vi "Halvorsen_2D_Lyapunov.vi"(11 "Initial Conditions":ext[](array[numeric])=[0.1, 0.0, 0.1]) -> ()   [LabVIEW 2016]
panel:
  out "Elapsed Time, s.":dbl
  out "Lyapunov":ext[][](graph)
  in  "Initial Conditions Inc":ext[](array[numeric])=[1e-10, 1e-10, 1e-10]
  in  "X_Inc":dbl[](array[numeric])=[0.02, 0.0, 0.0]
  in  "Final_X":dbl=0.35
  in  "Param_X":i32
  in  "Param_Y":i32=1
  in  "Final Y":dbl=0.35
  in  "Y_Inc":dbl[](array[numeric])=[0.0, 0.02, 0.0]
  in  "Parameter_Vector":ext[](array[numeric])=[0.01, 0.01, 0.1]
  out "Current_Param":ext[](array[numeric])=[0.01, 0.29000000000000000582, 0.1]
  in  "Время, с":ext=300.0
  in  "Hmin":ext=0.00099999999999999999996
  in  "Hmax":ext=1.0
  in  "tolerance":ext=1e-12
  in  "Шаг h, с":ext=0.01
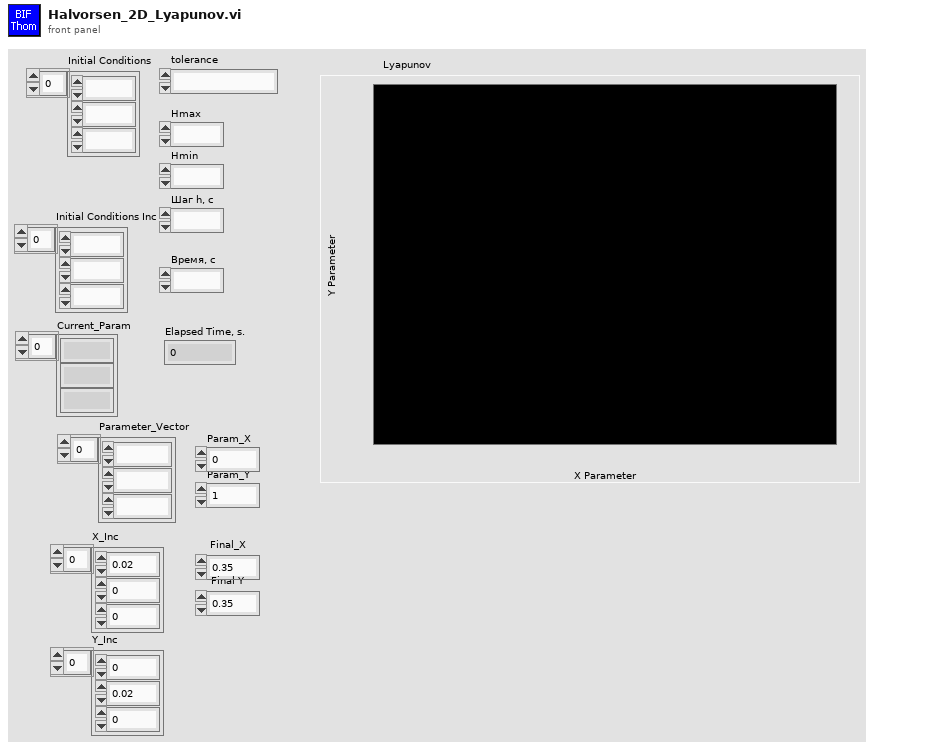
[diagram p1: front panel]
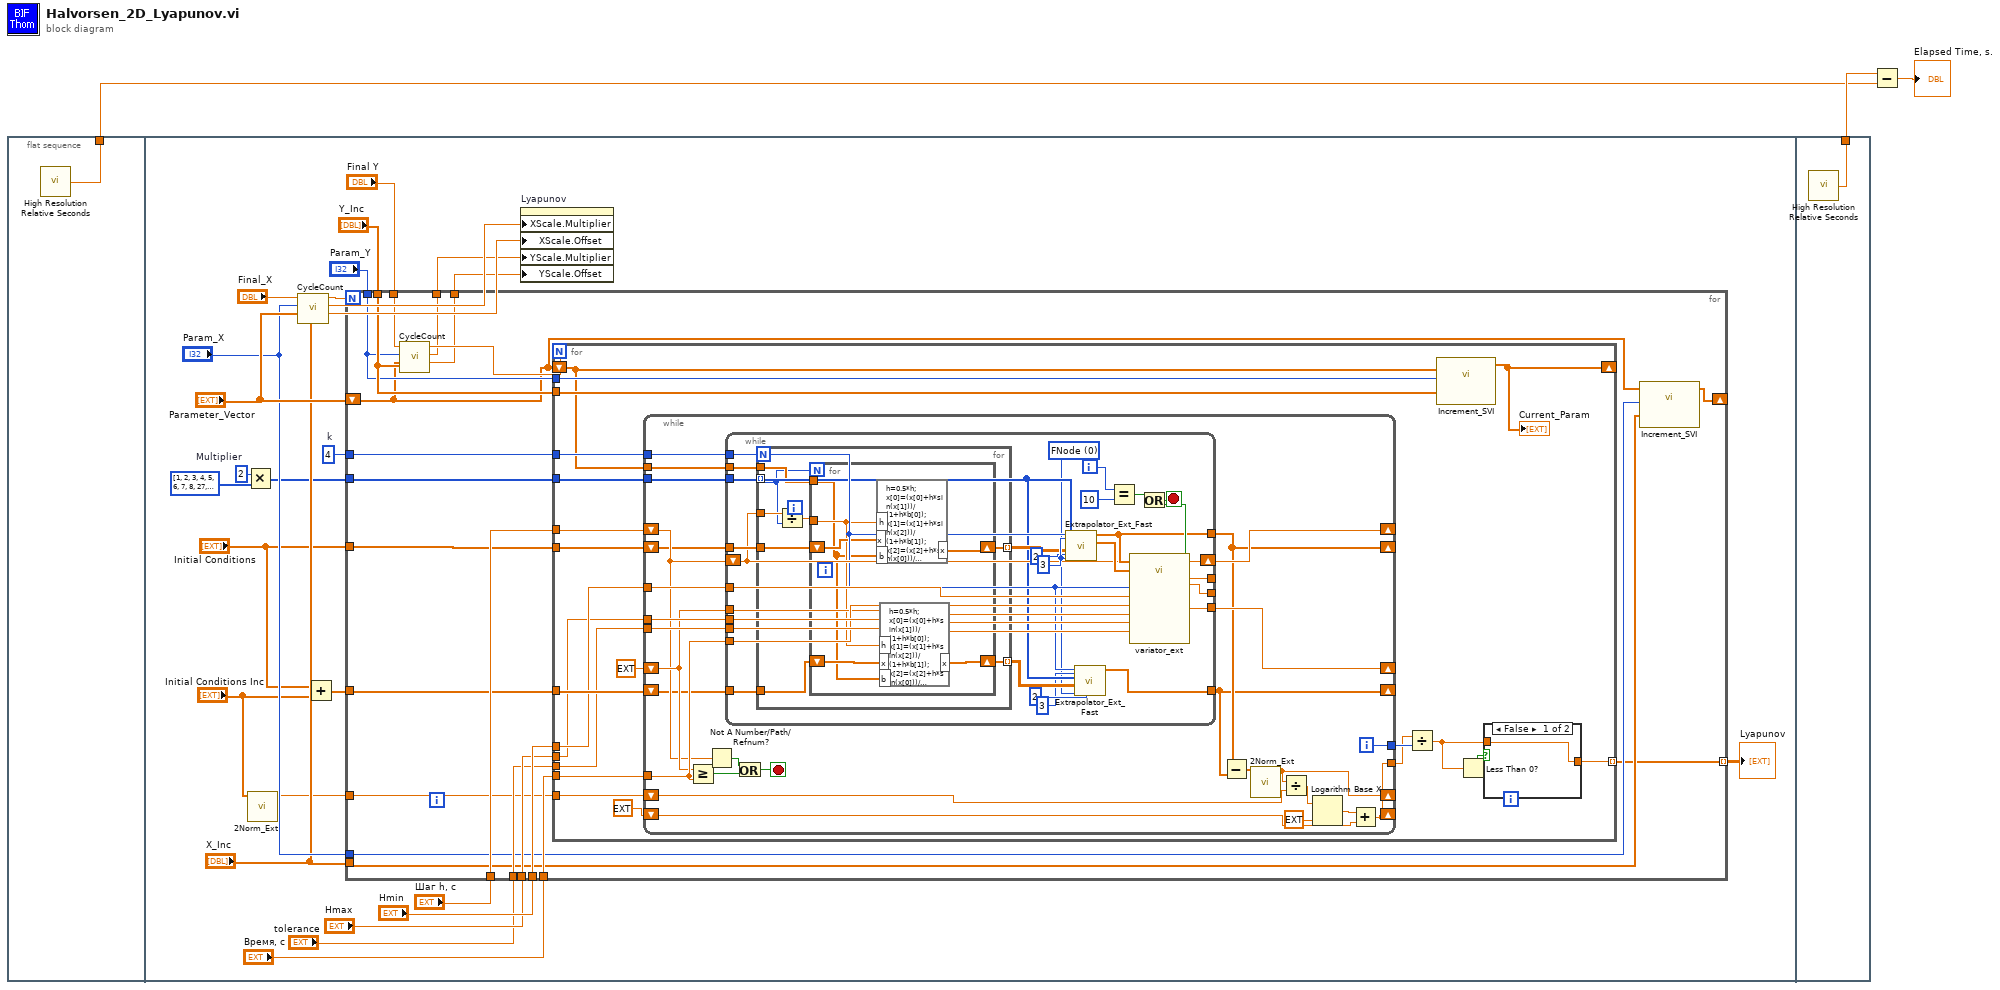
[diagram p0: block diagram]
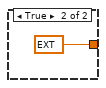
[diagram p2: hidden frame]
diagram:
  n1 = flat-sequence {
    tunnel: [w4] -> w2
    tunnel: [w145] -> w3
    frame #0 {
      n2 = call <vilib>:"High Resolution Relative Seconds.vi"() -> ("relative seconds"=w4:dbl)
    }
    frame #1 {
      w10 = 4  # k
      w17 = 2  # Multiplier
      n3 = Multiply(x=w17, y=i32[] [1, 2, 3, 4, 5, 6, 7, 8, 27, 30, 33] ("n")) -> (x*y=w15:i32[])
      n4 = call "2Norm_Ext.vi"("Input vector"="Initial Conditions Inc") -> ("2 Norm"=w13:ext)  [unwired: 10 in]
      n5 = call "CycleCount.vi"("Increment_Vector"="X_Inc", "Parameter_Vector"="Parameter_Vector", "Parameter Number"="Param_X", "Final_Parameter_Value"="Final_X") -> ("Parameter Offset"=w7:ext, "Parameter Multiplier"=w8:dbl, "Cycle Count"=w25:ext)  [unwired: 5 in]
      n6 = Add(x="Initial Conditions", y="Initial Conditions Inc") -> (x+y=w14:ext[])
      n7 = for {
        N: w25 -> [_]
        tunnel: "Шаг h, с" -> [w51]
        tunnel: "Initial Conditions" -> [w50]
        tunnel: "Hmin" -> [w49]
        tunnel: "Hmax" -> [w48]
        tunnel: "tolerance" -> [w47]
        tunnel: "Время, с" -> [w46]
        shift-right: [w34] -> _
        shift-left: "Parameter_Vector" -> [w36]
        tunnel: "Param_X" -> [w45]
        tunnel: "X_Inc" -> [w44]
        tunnel: "Final Y" -> [w43]
        tunnel: "Param_Y" -> [w40]
        tunnel: "Y_Inc" -> [w41]
        tunnel: w15 -> [w39]
        tunnel: w14 -> [w38]
        tunnel: [w37] -> w9 mode=indexing
        tunnel: w13 -> [w35]
        tunnel: w10 -> [w33]
        tunnel: [w32] -> w6
        tunnel: [w31] -> w5
        n8 = call "CycleCount.vi"("Increment_Vector"=w41, "Parameter_Vector"=w36, "Parameter Number"=w40, "Final_Parameter_Value"=w43) -> ("Parameter Offset"=w31:ext, "Parameter Multiplier"=w32:dbl, "Cycle Count"=w42:ext)  [unwired: 5 in]
        n9 = for {
          N: w42 -> [_]
          tunnel: w33 -> [w65]
          tunnel: w51 -> [w63]
          tunnel: w46 -> [w62]
          tunnel: w47 -> [w60]
          tunnel: w49 -> [w64]
          tunnel: w48 -> [w61]
          tunnel: w39 -> [w66]
          tunnel: w50 -> [w68]
          shift-right: [w71] -> _
          shift-left: w36 -> [w57]
          tunnel: w40 -> [w72]
          tunnel: w41 -> [w58]
          tunnel: w38 -> [w67]
          tunnel: [w53] -> w37 mode=indexing
          tunnel: w35 -> [w59]
          n10 = while {
            shift-right: [w79] -> _
            shift-left: w68 -> [w85]
            tunnel: w66 -> [w99]
            tunnel: w65 -> [w98]
            shift-right: [w94] -> _
            shift-left: w63 -> [w87]
            shift-right: [w91] -> _
            shift-left: ext 0.0 ("New time") -> [w92]
            tunnel: w62 -> [w93]
            tunnel: w60 -> [w95]
            tunnel: w64 -> [w97]
            tunnel: w61 -> [w96]
            tunnel: w57 -> [w90]
            shift-right: [w78] -> _
            shift-left: w67 -> [w73]
            shift-right: [w76] -> _
            shift-left: w59 -> [w80]
            shift-right: [w75] -> _
            shift-left: ext 0.0 -> [w81]
            tunnel: [w75] -> w55
            tunnel: [w74] -> w56
            i -> [w74]
            stop <- w89 stop-if-true
            n11 = Greater Or Equal?(x=w92, y=w93) -> (x >= y?=w88:bool)
            n12 = Not A Number/Path/Refnum?(number/path/refnum=w87) -> (NaN/Path/Refnum?=w86:bool)
            n13 = while {
              tunnel: w97 -> [w123]
              tunnel: w96 -> [w126]
              tunnel: w95 -> [w122]
              tunnel: w98 -> [w106]
              tunnel: w99 -> [w105]
              tunnel: w85 -> [w124]
              shift-right: [w117] -> w94
              shift-left: w87 -> [w109]
              tunnel: [w109] -> _
              tunnel: [w116] -> _
              tunnel: [w115] -> w79
              tunnel: w93 -> [w114]
              tunnel: w92 -> [w113]
              tunnel: [w111] -> w91
              tunnel: w90 -> [w110]
              tunnel: w73 -> [w107]
              tunnel: [w101] -> w78
              i -> [w112]
              stop <- w118 stop-if-true
              w100 = u16 0 items=["FNode", "MathScript", "ECD8 Arrays", "ECD8 Fnode", "ECD8 FnodeDiv"] ("Ext.Type")
              n14 = for {
                N: w106 -> [_]
                tunnel: w105 -> [w131] mode=indexing
                tunnel: w109 -> [w136]
                tunnel: w124 -> [w134]
                tunnel: [w135] -> w125 mode=indexing
                tunnel: w110 -> [w132]
                tunnel: w107 -> [w130]
                tunnel: [w129] -> w104 mode=indexing
                n15 = Divide(x=w136, y=w131) -> (x/y=w133:ext)
                n16 = for {
                  N: w131 -> [_]
                  shift-right: [w142] -> w135
                  shift-left: w134 -> [w141]
                  tunnel: w133 -> [w138]
                  tunnel: w132 -> [w137]
                  shift-right: [w140] -> w129
                  shift-left: w130 -> [w139]
                  n17 = formula code="h=0.5*h;\nx[0]=(x[0]+h*sin(x[1]))/(1+h*b[0]);\nx[1]=(x[1]+h*sin(x[2]))/(1+h*b[1]);\nx[2]=(x[2]+h*sin(x[0]))/(1+h*b[2]);\nx[2]=x[2]+h*(-b[2]*x[2]+sin(x[0]));\nx[1]=x[1]+h*(-b[1]*x[1]+sin(x[2]));\nx[0]=x[0]+h*(-b[0]*x[0]+sin(x[1]));"("x"=w141, "b"=w137, "h"=w138) -> ("x"=w142:ext[])
                  n18 = formula code="h=0.5*h;\nx[0]=(x[0]+h*sin(x[1]))/(1+h*b[0]);\nx[1]=(x[1]+h*sin(x[2]))/(1+h*b[1]);\nx[2]=(x[2]+h*sin(x[0]))/(1+h*b[2]);\nx[2]=x[2]+h*(-b[2]*x[2]+sin(x[0]));\nx[1]=x[1]+h*(-b[1]*x[1]+sin(x[2]));\nx[0]=x[0]+h*(-b[0]*x[0]+sin(x[1]));"("x"=w139, "b"=w137, "h"=w138) -> ("x"=w140:ext[])
                }
              }
              n19 = call "Extrapolator_Ext_Fast.vi"("Порядок экстраполятора"=2 ("Ext. Order"), "Dimension"=3 ("input variable"), "Ext.Type"=w100, "Х - нач. условия"=w125, "n"=w105, "k"=w106) -> ("TPrev"=w127:ext[], "Tout"=w115:ext[])  [unwired: 4 in]
              n20 = call "Extrapolator_Ext_Fast.vi"("Порядок экстраполятора"=2 ("Ext. Order"), "Dimension"=3 ("input variable"), "Ext.Type"=w100, "Х - нач. условия"=w104, "n"=w105, "k"=w106) -> ("Tout"=w101:ext[])  [unwired: 4 in, 1 out]
              n21 = Equal?(x=w112, y=10) -> (x = y?=w120:bool)
              n22 = call "variator_ext.vi"("Tout"=w115, "tolerance"=w122, "Hmax"=w126, "TPrev"=w127, "Шаг h, с"=w109, "Current time"=w113, "k"=w106, "Hmin"=w123, "tmax"=w114) -> ("Hnew"=w117:ext, "error estimation"=w116:ext, "New time"=w111:ext, "stop"=w119:bool)  [unwired: 3 in]
              n23 = Or(x=w120, y=w119) -> (x .or. y?=w118:bool)
            }
            n24 = Or(x=w86, y=w88) -> (x .or. y?=w89:bool)
            n25 = Subtract(x=w79, y=w78) -> (x-y=w77:ext[])
            n26 = call "2Norm_Ext.vi"("Input vector"=w77) -> ("2 Norm"=w76:ext)  [unwired: 10 in]
            n27 = Divide(x=w76, y=w80) -> (x/y=w84:ext)
            n28 = Logarithm Base X(1:ext 10.0 ("x"), 2:w84) -> (0:w83:ext)
            n29 = Add(x=w83, y=w81) -> (x+y=w75:ext)
          }
          n30 = Divide(x=w55, y=w56) -> (x/y=w52:ext)
          n31 = call "Increment_SVI.vi"("Increment_Vector"=w58, "Param_Index"=w72, "Parameter_Vector"=w57) -> ("Parameters_Out"=w71:ext[])  [unwired: 7 in, 1 out]
          "Current_Param" <- w71
          n32 = Less Than 0?(x=w52) -> (x < 0?=w54:bool)
          n33 = case shown="False" w54 {
            tunnel: [w143 ext 1e-8] -> w53
            tunnel: w52 -> [w143 _]
            frame False {
            }
            frame True {
            }
          }
        }
        n34 = call "Increment_SVI.vi"("Increment_Vector"=w44, "Param_Index"=w45, "Parameter_Vector"=w36) -> ("Parameters_Out"=w34:ext[])  [unwired: 7 in, 1 out]
      }
      "Lyapunov" <- w9
      n35 = property on="Lyapunov" class="IntGraph (strict)"("XScale.Multiplier"=w8, "XScale.Offset"=w7, "YScale.Multiplier"=w6, "YScale.Offset"=w5) -> ()  [unwired: 2 in, 2 out]
    }
    frame #2 {
      n36 = call <vilib>:"High Resolution Relative Seconds.vi"() -> ("relative seconds"=w145:dbl)
    }
  }
  n37 = Subtract(x=w3, y=w2) -> (x-y=→"Elapsed Time, s.":dbl)
